vi "VISA Make Info.vi"(1 "prefix":string, 2 "Use serial cfg parameters (False)":bool, 3 "serial cfg":T1={"Baud rate"=9600, "Data bits"=8, "Parity"=0, "Stop bits"=10, "Flow control"=0, "End Mode Read"=enum."None", "End Mode Write"=enum."None", "Term character"=0, "Term enable"=FALSE} {"Flow control" items=["None", "XON/XOFF", "CTS/RTS", "XON/XOFF + CTS/RTS", "DTR/DSR", "XON/XOFF + DTR/DSR"]; "Stop bits" items=["1 bit"=10, "1.5 bits"=15, "2 bits"=20]; "Parity" items=["None", "Odd", "Even", "Mark", "Space"]; "Data bits" items=["5 bits"=5, "6 bits"=6, "7 bits"=7, "8 bits"=8]; "Baud rate" items=["150 Bd"=150, "300 Bd"=300, "600 Bd"=600, "1200 Bd"=1200, "2400 Bd"=2400, "4800 Bd"=4800, "9600 Bd"=9600, "19.2 kBd"=19200, "38.4 kBd"=38400, "57.6 kBd"=57600, "115.2 kBd"=115200]}, 4 "VISA in":refnum<visa-resource-name>) -> (0 "info string":string)   [LabVIEW 2020]
doc: "Makes information string with bus address and bus setup if available.\nNote serial parameters reverts to some default after VISA close, so they must be fed using serial cfg!"
uses:
  met_serial_setup.ctl
panel:
  in  "Serial Settings:Parity":u16(ring) items=["None", "Odd", "Even", "Mark", "Space"]
  in  "Serial Settings:Flow Control":u16(ring) items=["None", "XON/XOFF", "RTS/CTS", "XON/XOFF & RTS/CTS", "DTR/DSR", "XON/XOFF & DTR/DSR"]
  in  "Serial Settings:End Mode for Reads":u16(ring) items=["None", "Last Bit", "TermChar"]
  out "Interface Information:Interface Description":string
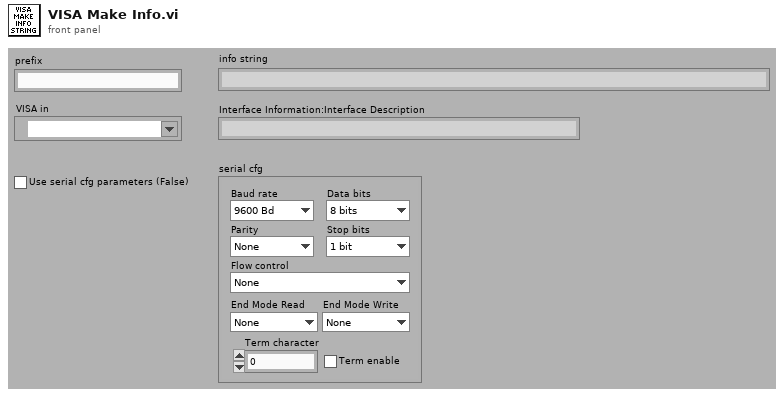
[diagram p1: front panel]
types:
  T1 = typedef "met_serial_setup.ctl" = cluster{"Baud rate":i32, "Data bits":i32, "Parity":i32, "Stop bits":i32, "Flow control":i32, "End Mode Read":enum16{"None", "Last Bit", "TermChar"}, "End Mode Write":enum16{"None", "Last Bit", "TermChar"}, "Term character":u8, "Term enable":bool}
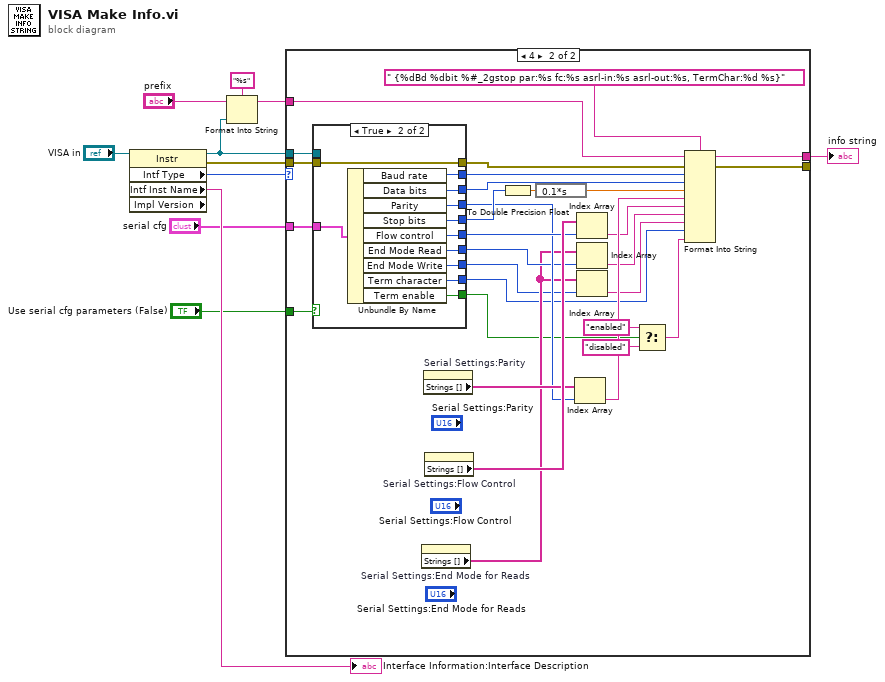
[diagram p0: block diagram]
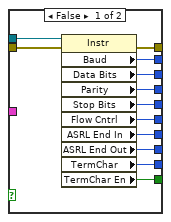
[diagram p3: hidden frame]
diagram:
  n1 = property class="Instr" props=["Intf Type", "Intf Inst Name", "Impl Version"](reference="VISA in") -> (reference out=w6:refnum<visa-resource-name>, error out=w4:errorcluster, "Intf Type"=w9:u16, "Intf Inst Name"=→"Interface Information:Interface Description":string)  [unwired: 1 in, 1 out]
  n2 = Format Into String(format string="%s", initial string="prefix", w6) -> (resulting string=w3:string)  [unwired: 1 in, 1 out]
  n3 = case shown="4" w9 {
    tunnel: w6 -> [_ w43]
    tunnel: [w12 w23] -> w8
    tunnel: w4 -> [w13 w22]
    tunnel: [w13 w20] -> _
    tunnel: w3 -> [w12 w19]
    tunnel: "Use serial cfg parameters (False)" -> [_ w15]
    tunnel: "serial cfg" -> [_ w14]
    frame 0, Default {
    }
    frame 4 {
      n4 = case shown="True" w15 {
        tunnel: w43 -> [w55 _]
        tunnel: [w54 w64] -> w41
        tunnel: [w53 w63] -> w40
        tunnel: [w52 w61] -> w39
        tunnel: [w51 w60] -> w37
        tunnel: [w50 w62] -> w35
        tunnel: [w49 w59] -> w32
        tunnel: [w48 w58] -> w30
        tunnel: [w47 w57] -> w28
        tunnel: [w46 w56] -> w26
        tunnel: w22 -> [w45 w65]
        tunnel: [w44 w65] -> w21
        tunnel: w14 -> [_ w66]
        frame False {
          n5 = property class="Instr"(reference=w55, error in=w45) -> (error out=w44:errorcluster, "Baud"=w54:u32, "Data Bits"=w53:u16, "Parity"=w50:u16, "Stop Bits"=w52:u16, "Flow Cntrl"=w51:u16, "ASRL End In"=w49:u16, "ASRL End Out"=w48:u16, "TermChar"=w47:u8, "TermChar En"=w46:bool)  [unwired: 1 out]
        }
        frame True {
          n6 = Unbundle By Name(w66) -> ("Baud rate"=w64:i32, "Data bits"=w63:i32, "Parity"=w62:i32, "Stop bits"=w61:i32, "Flow control"=w60:i32, "End Mode Read"=w59:enum16{"None", "Last Bit", "TermChar"}, "End Mode Write"=w58:enum16{"None", "Last Bit", "TermChar"}, "Term character"=w57:u8, "Term enable"=w56:bool)
        }
      }
      n7 = property on="Serial Settings:End Mode for Reads" class="Ring (strict)"() -> ("Strings []"=w31:string[])  [unwired: 2 in, 2 out]
      n8 = property on="Serial Settings:Parity" class="Ring (strict)"() -> ("Strings []"=w36:string[])  [unwired: 2 in, 2 out]
      n9 = property on="Serial Settings:Flow Control" class="Ring (strict)"() -> ("Strings []"=w38:string[])  [unwired: 2 in, 2 out]
      n10 = To Double Precision Float(number=w39) -> (double precision float=w17:dbl)
      n11 = expression code="0.1*s"(w17) -> (w18:dbl)
      n12 = Index Array(array=w36, index=w35) -> (element=w34:string)
      n13 = Index Array(array=w38, index=w37) -> (element=w33:string)
      n14 = Index Array(array=w31, index=w32) -> (element=w16:string)
      n15 = Index Array(array=w31, index=w30) -> (element=w29:string)
      n16 = Select(t="enabled", s=w26, f="disabled") -> (s? t:f=w27:string)
      n17 = Format Into String(format string=" {%dBd %dbit %#_2gstop par:%s fc:%s asrl-in:%s asrl-out:%s, TermChar:%d %s}", initial string=w19, error in=w21, w41, w40, w18, w34, w33, w16, w29, w28, w27) -> (resulting string=w23:string, error out=w20:errorcluster)
    }
  }
  "info string" <- w8
